vi "Function_Flash Detection #.vi"(8 "Error in":errorcluster, 9 "CoordSys In":T1 {"Measurement System"."Axis Reference" items=["Direct", "Indirect"]; "Measurement System"."Angle (deg)" format="%.2f"; "Measurement System"."Origin"."Y" format="%.2f"; "Measurement System"."Origin"."X" format="%.2f"; "Reference System"."Axis Reference" items=["Direct", "Indirect"]; "Reference System"."Angle (deg)" format="%.2f"; "Reference System"."Origin"."Y" format="%.2f"; "Reference System"."Origin"."X" format="%.2f"}, 10 "Data Cluster In":cluster{"Name":string, "Variant In":variant}, 11 "Image Dst In":T3) -> (0 "Error out":errorcluster, 1 "Perpendicular Line(Offset)":T2, 2 "Fit Line(Offset)":T2, 3 "Result(Flash)":cluster{"Name":string, "NG?":bool, "Score":dbl}, 4 "Time":u32)   [LabVIEW 2013]
uses:
  <vilib>/vision/Image Controls.llb/IMAQ Image.ctl
  Control/Control_Flash Detection Setting.ctl
  <vilib>/vision/Measure.llb/Edge Options.ctl
  <vilib>/vision/Measure.llb/Edge Polarity.ctl
  <vilib>/vision/NI_Vision_Development_Module.lvlib
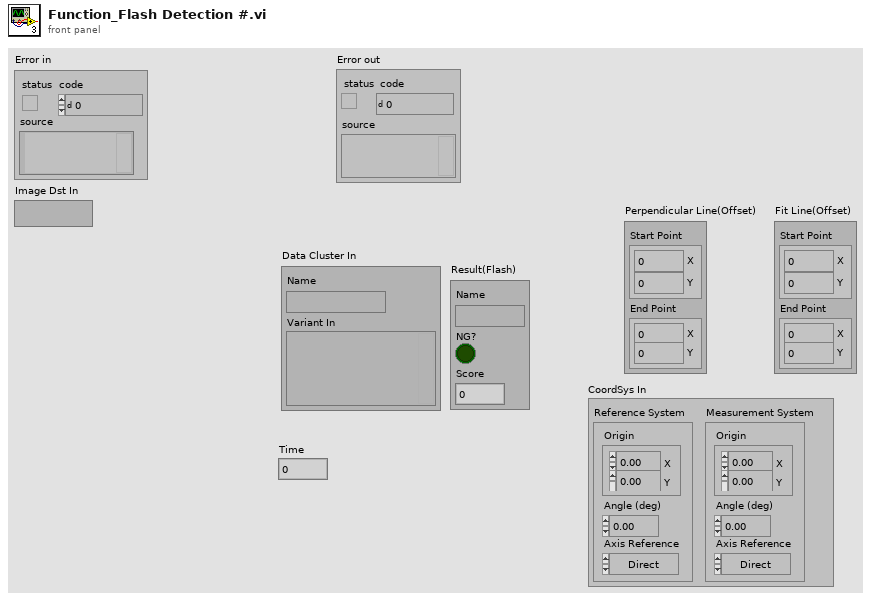
[diagram p1: front panel]
types:
  T1 = typedef "IMAQ Coordinate System" = cluster{"Reference System":cluster{"Origin":cluster{"X":sgl, "Y":sgl}, "Angle (deg)":sgl, "Axis Reference":u32}, "Measurement System":cluster{"Origin":cluster{"X":sgl, "Y":sgl}, "Angle (deg)":sgl, "Axis Reference":u32}}
  T2 = cluster{"Start Point":cluster{"X":i32, "Y":i32}, "End Point":cluster{"X":i32, "Y":i32}}
  T3 = typedef "IMAQ Image.ctl" = refnum<image>
  T4 = typedef "Control_Flash Detection Setting.ctl" = cluster{"Name":string, "ROI":cluster{"Global Rectangle":i32[], "Contours":cluster{"ID":enum32{"External", "Internal"}, "Type":u32, "Coordinates":i32[]}[]}, "Image Process":cluster{"Image Process":bool, "Method":enum32{"Differentiation", "Gradient", "Prewitt", "Roberts", "Sigma", "Sobel"}, "Kernel Size":i32, "Divider":sgl}, "Edge Setting(毛邊)":cluster{"Edge Options":T5, "Flash Detection":enum16{"Datum C", "Arc"}, "Scan Direction":u16, "Step Size":i32}, "條件(毛邊)":cluster{"毛邊長度":dbl}}
  T5 = typedef "Edge Options.ctl" = cluster{"Edge Polarity":T6, "Kernel Size":u32, "Width":u32, "Minimum Edge Strength":sgl, "Interpolation Type":enum32{"Zero Order", "Bilinear", "Quadratic", "Cubic", "Bilinear Fixed"}, "Data Processing Method":enum32{"Average", "Median"}}
  T6 = typedef "Edge Polarity.ctl" = u32
  T7 = cluster{"Global Rectangle":i32[], "Contours":cluster{"ID":enum32{"External", "Internal"}, "Type":u32, "Coordinates":i32[]}[]}
  T8 = cluster{"Image Process":bool, "Method":enum32{"Differentiation", "Gradient", "Prewitt", "Roberts", "Sigma", "Sobel"}, "Kernel Size":i32, "Divider":sgl}
  T9 = cluster{"Edge Options":T5, "Flash Detection":enum16{"Datum C", "Arc"}, "Scan Direction":u16, "Step Size":i32}
  T10 = cluster{"Origin":cluster{"X":sgl, "Y":sgl}, "Angle (deg)":sgl, "Axis Reference":u32}
  T11 = typedef "ROI Descriptor" = cluster{"Global Rectangle":i32[], "Contours":cluster{"ID":enum32{"External", "Internal"}, "Type":u32, "Coordinates":i32[]}[]}
  T12 = enum32{"Differentiation", "Gradient", "Prewitt", "Roberts", "Sigma", "Sobel"}
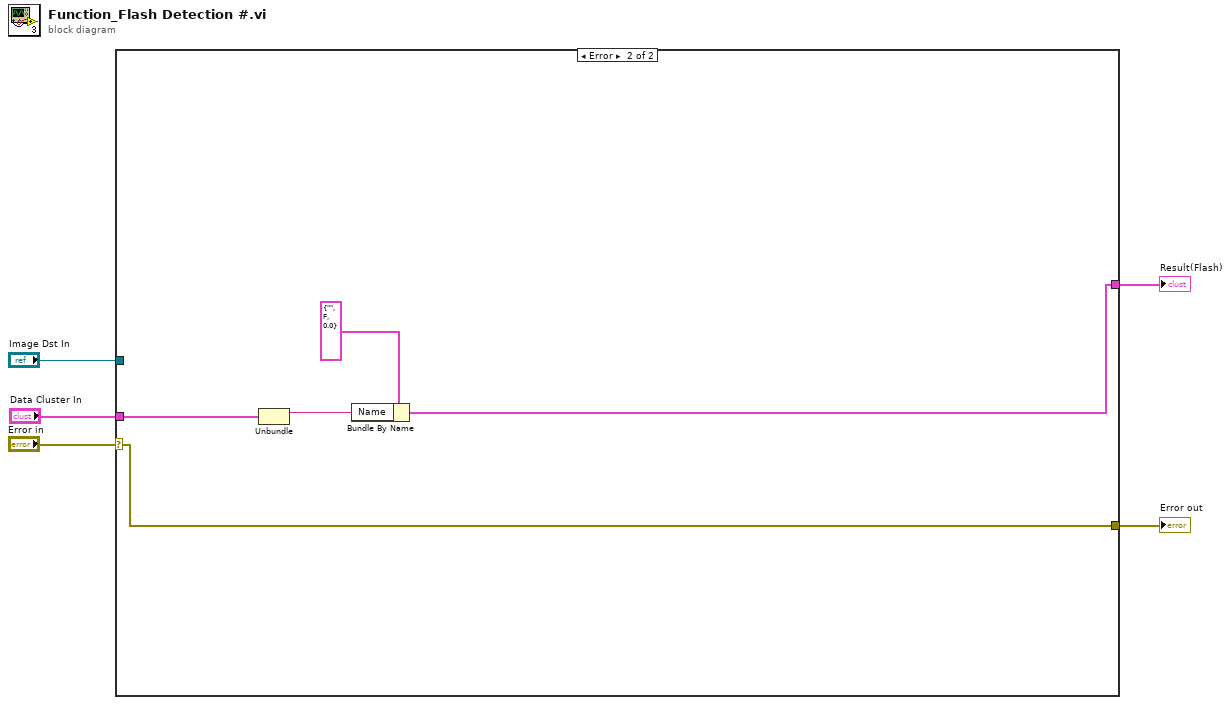
[diagram p0: block diagram]
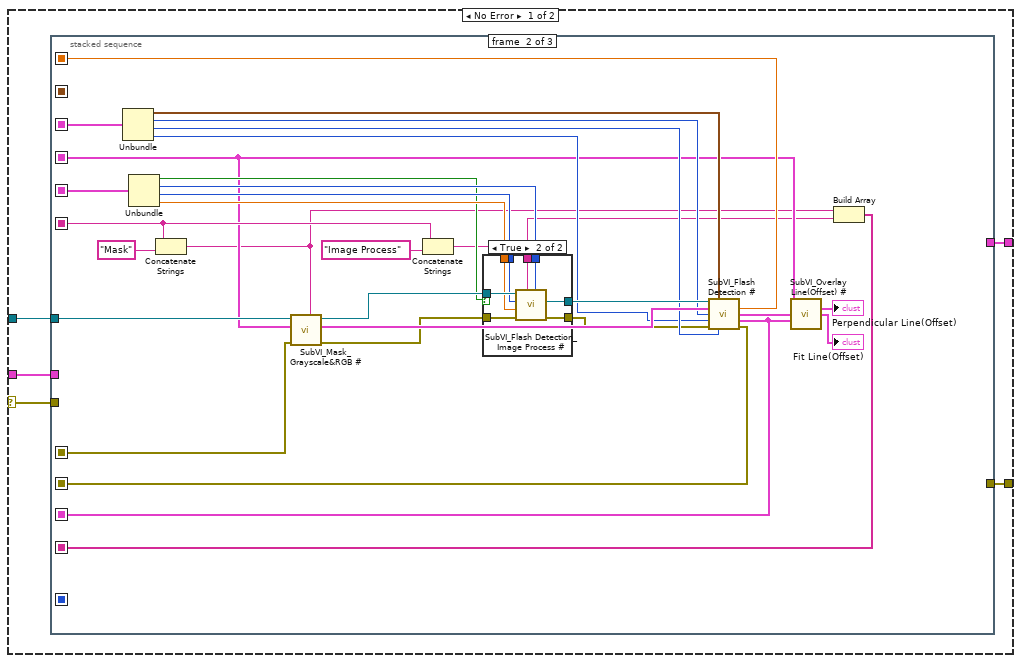
[diagram p2: hidden frame]
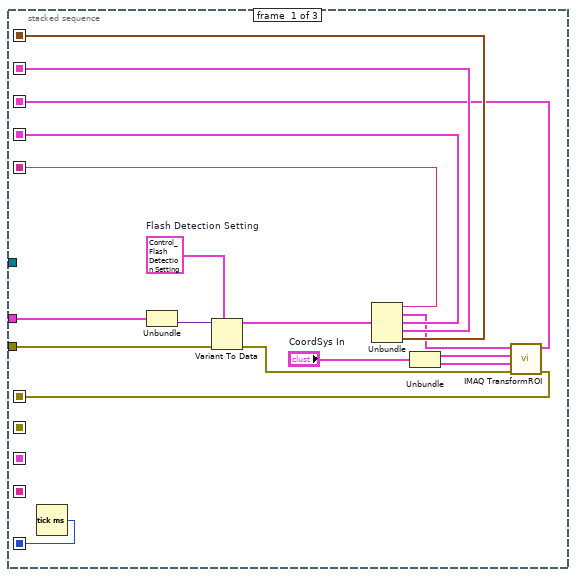
[diagram p3: hidden frame]
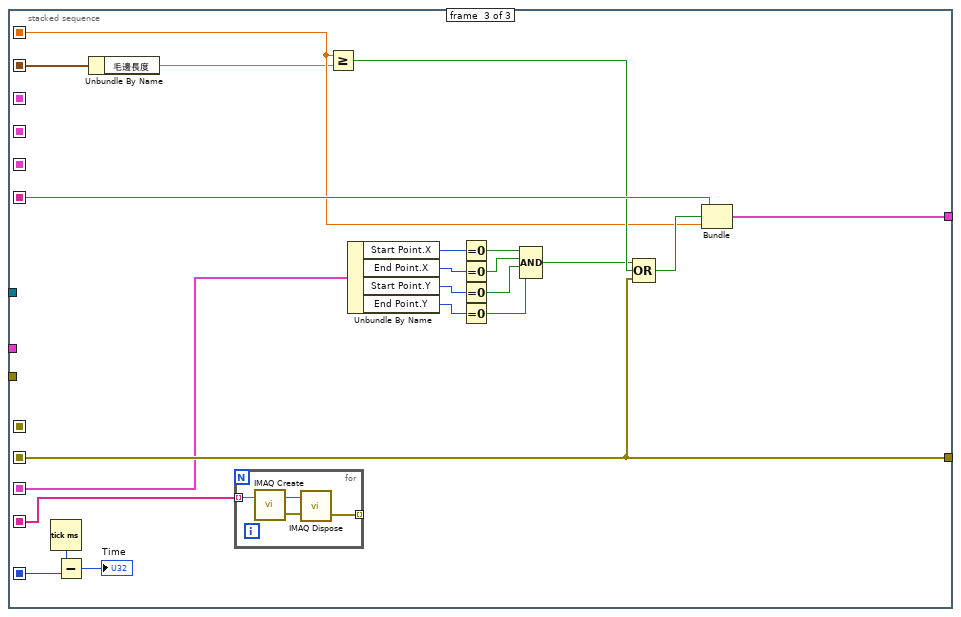
[diagram p5: hidden frame]
diagram:
  n1 = case shown="Error" "Error in" {
    selector: "Error in" -> [w7 w98]
    tunnel: "Image Dst In" -> [w10 _]
    tunnel: [w9 w98] -> w4
    tunnel: [w8 w94] -> w3
    tunnel: "Data Cluster In" -> [w6 w95]
    frame No Error {
      n2 = stacked-sequence {
        seq-local: [w25 _ _] -> [_ w50 w84]
        seq-local: [w20 _ _] -> [_ w52 _]
        seq-local: [w14 _ _] -> [_ w35 _]
        seq-local: [w24 _ _] -> [_ w53 _]
        seq-local: [w23 _ _] -> [_ _ w87]
        seq-local: [w19 _ _] -> [_ _ w80]
        seq-local: [_ w38 _] -> [_ _ w82]
        seq-local: [_ w37 _] -> [_ _ w85]
        seq-local: [_ w28 _] -> [_ _ w77]
        seq-local: [w12 _ _] -> [_ w32 _]
        seq-local: [_ w29 _] -> [_ _ w78]
        tunnel: w7 -> [w21 _ _]
        tunnel: w10 -> [_ w46 _]
        tunnel: [_ _ w85] -> w9
        tunnel: [_ _ w81] -> w8
        tunnel: w6 -> [w11 _ _]
        frame #0 {
          w22 = T4 {"Name"="", "ROI"={"Global Rectangle"=[], "Contours"=[]}, "Image Process"={"Image Process"=FALSE, "Method"=enum."Differentiation", "Kernel Size"=0, "Divider"=0.0}, "Edge Setting(毛邊)"={"Edge Options"={"Edge Polarity"=0, "Kernel Size"=0, "Width"=0, "Minimum Edge Strength"=0.0, "Interpolation Type"=enum."Zero Order", "Data Processing Method"=enum."Average"}, "Flash Detection"=enum."Datum C", "Scan Direction"=0, "Step Size"=0}, "條件(毛邊)"={"毛邊長度"=0.0}}  # Flash Detection Setting
          n3 = Tick Count (ms)() -> (millisecond timer value=w23:u32)
          n4 = Unbundle(w11) -> ("Variant In"=w26:variant)  [unwired: 1 out]
          n5 = Variant To Data(error in=w21, type=w22, Variant=w26) -> (data=w27:T4, error out=w13:errorcluster)
          n6 = Unbundle(w27) -> ("Name"=w25:string, "ROI"=w15:T7, "Image Process"=w20:T8, "Edge Setting(毛邊)"=w24:T9, "條件(毛邊)"=w19:cluster{"毛邊長度":dbl})
          n7 = Unbundle("CoordSys In") -> ("Reference System"=w17:T10, "Measurement System"=w16:T10)
          n8 = call "IMAQ TransformROI"("error in (no error)"=w13, "New Reference"=w16, "Base Reference"=w17, "ROI Descriptor"=w15) -> ("error out"=w12:errorcluster, "ROI Descriptor out"=w14:T11)  [unwired: 6 in]
        }
        frame #1 {
          n9 = Unbundle(w53) -> ("Edge Options"=w45:T5, "Flash Detection"=w44:enum16{"Datum C", "Arc"}, "Scan Direction"=w43:u16, "Step Size"=w39:i32)
          n10 = Unbundle(w52) -> ("Image Process"=w40:bool, "Method"=w49:T12, "Kernel Size"=w48:i32, "Divider"=w47:sgl)
          n11 = Concatenate Strings(w50, "Mask" ("string")) -> (w31:string)
          n12 = call "SubVI_Mask_Grayscale&RGB #.vi"("Image Register Name"=w31, "Error in"=w32, "ROI Descriptor"=w35, "Image Src In"=w46) -> ("Error out"=w42:errorcluster, "ROI Descriptor out"=w55:T11, "Image Dst Out"=w54:T3)  [unwired: 4 in, 1 out]
          n13 = Concatenate Strings(w50, "Image Process" ("string")) -> (w30:string)
          n14 = case shown="True" w40 {
            tunnel: [w59 w67] -> w56
            tunnel: w54 -> [w59 w66]
            tunnel: w30 -> [_ w65]
            tunnel: w49 -> [_ w64]
            tunnel: w48 -> [_ w63]
            tunnel: w47 -> [_ w62]
            tunnel: w42 -> [w58 w61]
            tunnel: [w58 w60] -> w41
            frame False {
            }
            frame True {
              n15 = call "SubVI_Flash Detection_Image Process #.vi"("Method"=w64, "Image Register Name"=w65, "Error in"=w61, "Divider"=w62, "Kernel Size"=w63, "Image Src In"=w66) -> ("Error out"=w60:errorcluster, "Image Dst Out"=w67:T3)  [unwired: 3 in, 1 out]
            }
          }
          n16 = call "SubVI_Flash Detection #.vi"("Image In"=w56, "Edge Options"=w45, "ROI Descriptor"=w55, "Flash Detection"=w44, "Step Size"=w39, "Error in"=w41, "Scan Direction"=w43) -> ("Distance"=w38:dbl, "Perpendicular Line"=w36:T2, "Fit Line"=w28:T2, "Error out"=w37:errorcluster)  [unwired: 4 in, 1 out]
          n17 = call "SubVI_Overlay Line(Offset) #.vi"("ROI Descriptor"=w35, "Perpendicular Line"=w36, "Fit Line"=w28) -> ("Perpendicular Line(Offset)"=→"Perpendicular Line(Offset)":T2, "Fit Line(Offset)"=→"Fit Line(Offset)":T2)  [unwired: 11 in]
          n18 = Build Array(w31, w30) -> (w29:string[])
        }
        frame #2 {
          n19 = Tick Count (ms)() -> (millisecond timer value=w89:u32)
          n20 = Subtract(x=w89, y=w87) -> (x-y=→"Time":u32)
          n21 = Unbundle By Name(w80) -> ("毛邊長度"=w79:dbl)
          n22 = for {
            tunnel: w78 -> [w93] mode=indexing
            tunnel: [w90] -> _ mode=indexing
            n23 = call "IMAQ Create"("Image Name"=w93) -> ("New Image"=w92:T3, "error out"=w91:errorcluster)  [unwired: 4 in]
            n24 = call "IMAQ Dispose"("Image"=w92, "error in (no error)"=w91) -> ("error out"=w90:errorcluster)  [unwired: 4 in]
          }
          n25 = Greater Or Equal?(x=w82, y=w79) -> (x >= y?=w83:bool)
          n26 = Unbundle By Name(w77) -> ("Start Point.X"=w76:i32, "End Point.X"=w75:i32, "Start Point.Y"=w74:i32, "End Point.Y"=w73:i32)
          n27 = Equal To 0?(x=w76) -> (x = 0?=w72:bool)
          n28 = Equal To 0?(x=w75) -> (x = 0?=w71:bool)
          n29 = Equal To 0?(x=w74) -> (x = 0?=w70:bool)
          n30 = Equal To 0?(x=w73) -> (x = 0?=w69:bool)
          n31 = Compound Arithmetic op=AND(w72, w71, w70, w69) -> (w68:bool)
          n32 = Compound Arithmetic op=OR(w68, w83, w85) -> (w86:bool)
          n33 = Bundle("Name"=w84, w86, "Distance"=w82) -> (w81:cluster{"Name":string, bool, "Distance":dbl})  [unwired: 1 in]
        }
      }
    }
    frame Error {
      n34 = Unbundle(w95) -> ("Name"=w96:string)  [unwired: 1 out]
      n35 = Bundle By Name(cluster=cluster{"Name":string, bool, "Radius":dbl} {"Name"="", FALSE, "Radius"=0.0}, "Name"=w96) -> (w94:cluster{"Name":string, bool, "Radius":dbl})
    }
  }
  "Error out" <- w4
  "Result(Flash)" <- w3
